vi "Get Category.vi"(8 "error in (no error)":errorcluster, 11 "OPC UA Client editor node in":refnum<class "OPC UA Client editor node.lvclass">) -> (0 "error out":errorcluster, 2 "Category":string, 3 "OPC UA Client editor node out":refnum<class "OPC UA Client editor node.lvclass">)   [LabVIEW 2014, in "OPC UA Client editor node.lvclass"]
uses:
  OPC UA Client editor node.lvclass
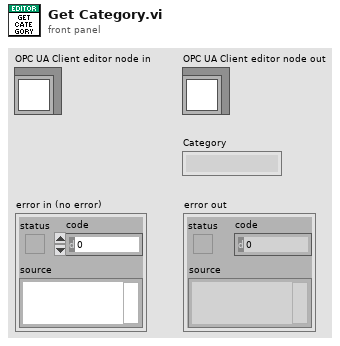
[diagram p1: front panel]
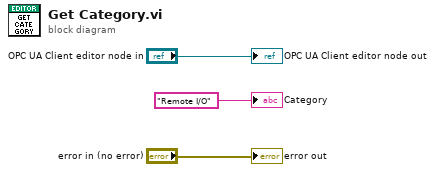
[diagram p0: block diagram]
diagram:
  "error out" <- "error in (no error)"
  "OPC UA Client editor node out" <- "OPC UA Client editor node in"
  "Category" <- "Remote I/O" ("Category")
